vi "Write Roles.vi"(8 "error in (no error)":errorcluster, 10 "Roles":T1, 11 "IndirectEnemyPlay in":refnum<class "IndirectEnemyPlay.lvclass">) -> (0 "error out":errorcluster, 3 "IndirectEnemyPlay out":refnum<class "IndirectEnemyPlay.lvclass">)   [LabVIEW 2023, in "IndirectEnemyPlay.lvclass"]
uses:
  IndirectEnemyPlay.lvclass
  AttackerBlockRole_class/AttackerBlockRole.lvclass
  MarkerRole_class/MarkerRole.lvclass
  IndirectEnemyPlay.lvclass/IndirectEnemyPlay.ctl
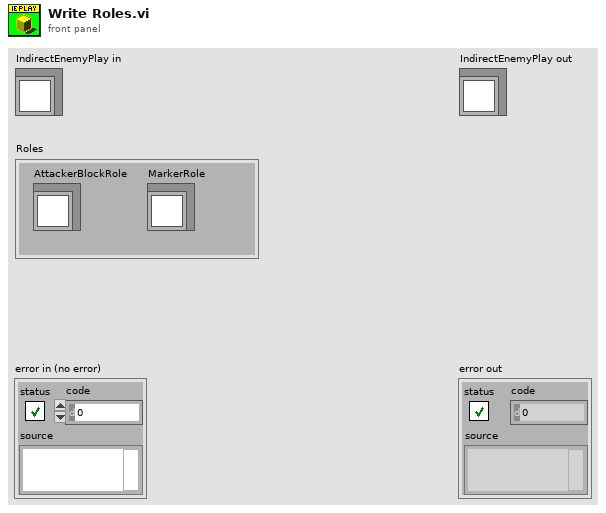
[diagram p1: front panel]
types:
  T1 = cluster{"AttackerBlockRole":refnum<class "AttackerBlockRole.lvclass">, "MarkerRole":refnum<class "MarkerRole.lvclass">}
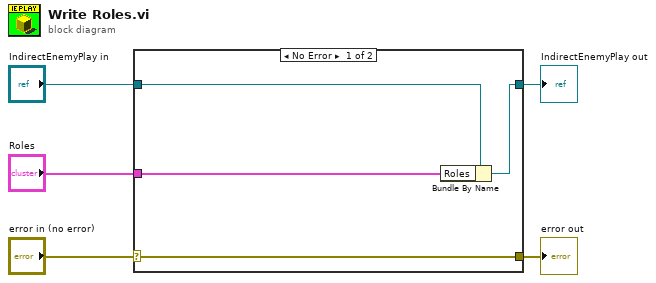
[diagram p0: block diagram]
diagram:
  n1 = case shown="No Error" "error in (no error)" {
    selector: "error in (no error)" -> [w9 w10]
    tunnel: [w9 w10] -> w4
    tunnel: [w7 w11] -> w2
    tunnel: "IndirectEnemyPlay in" -> [w8 w11]
    tunnel: "Roles" -> [w6 _]
    frame No Error {
      n2 = Bundle By Name(cluster=w8, "Roles"=w6) -> (w7:refnum<class "IndirectEnemyPlay.lvclass">)
    }
    frame Error {
    }
  }
  "error out" <- w4
  "IndirectEnemyPlay out" <- w2
